vi "Taiko_LHDataToStrArray.vi"(11 "LHData":T2={"SerNo"=1034578, "Features"=16974033, "FreqMin"=1, "FreqMax"=100000000, "CwPowerMax"=77500000, "PulsePowerMax"=14500000, "WavelengthNominal"=6400, "CaseTempMax"=700, "Protection"=TRUE, "LHTypeCtrlVoltage"=4085, "LHMaxVoltage"=3590, "CurrentTEP12V"=100, "LaserType"=16, "LHVersion"={"Major"=0, "Minor"=0}, "CalWarrentHours"=1000} {"LaserType" items=["UNDEFINED"=0, "LDH"=16, "LDH_FSL"=24, "LED"=32, "TA_SHG"=48, "FIBER"=64, "FIBER_FSL"=72, "FA"=80, "FA_SHG"=96, "BRIDGE"=240]}) -> (3 "StrArray":string[](array[string]))   [LabVIEW 2019]
uses:
  <userlib>/TaikoLaser/PDLM_LHData.ctl
  <userlib>/TaikoLaser/PDLM_LHData_LaserType.ctl
  <userlib>/TaikoLaser/PDLM_LHVersion.ctl
panel:
  out "LaserType":T1 items=["UNDEFINED"=0, "LDH"=16, "LDH_FSL"=24, "LED"=32, "TA_SHG"=48, "FIBER"=64, "FIBER_FSL"=72, "FA"=80, "FA_SHG"=96, "BRIDGE"=240]
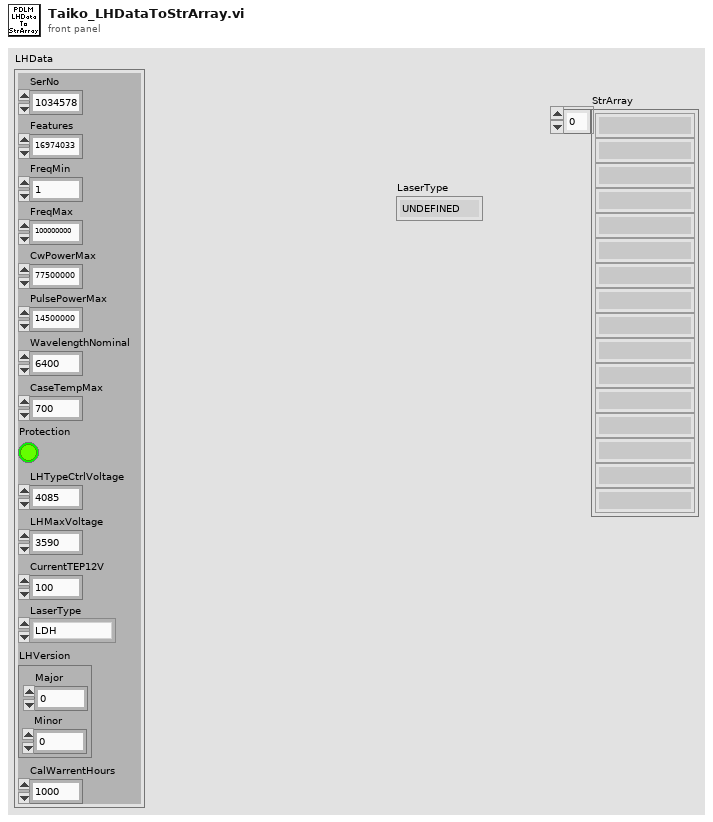
[diagram p1: front panel]
types:
  T1 = typedef "PDLM_LHData_LaserType.ctl" = u16
  T2 = typedef "PDLM_LHData.ctl" = cluster{"SerNo":u32, "Features":u32, "FreqMin":u32, "FreqMax":u32, "CwPowerMax":u32, "PulsePowerMax":u32, "WavelengthNominal":u16, "CaseTempMax":u16, "Protection":bool, "LHTypeCtrlVoltage":u16, "LHMaxVoltage":u16, "CurrentTEP12V":u16, "LaserType":T1, "LHVersion":T3, "CalWarrentHours":u16}
  T3 = typedef "PDLM_LHVersion.ctl" = cluster{"Major":u16, "Minor":u16}
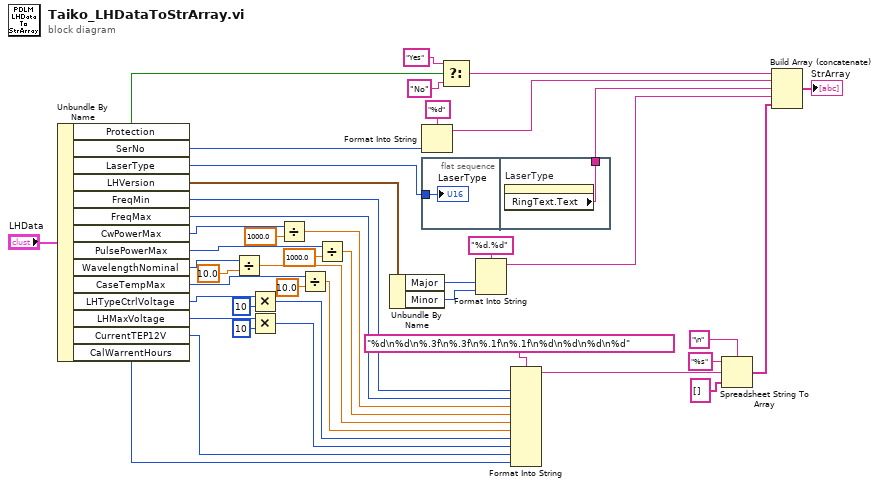
[diagram p0: block diagram]
diagram:
  n1 = Unbundle By Name("LHData") -> ("Protection"=w43:bool, "SerNo"=w40:u32, "LaserType"=w39:T1, "LHVersion"=w34:T3, "FreqMin"=w29:u32, "FreqMax"=w28:u32, "CwPowerMax"=w18:u32, "PulsePowerMax"=w14:u32, "WavelengthNominal"=w11:u16, "CaseTempMax"=w8:u16, "LHTypeCtrlVoltage"=w5:u16, "LHMaxVoltage"=w2:u16, "CurrentTEP12V"=w27:u16, "CalWarrentHours"=w26:u16)
  n2 = Divide(x=w11, y=10.0) -> (x/y=w10:dbl)
  n3 = Multiply(x=w5, y=u16 10) -> (x*y=w4:u16)
  n4 = Multiply(x=w2, y=u16 10) -> (x*y=w1:u16)
  n5 = Divide(x=w18, y=1000.0) -> (x/y=w16:dbl)
  n6 = Divide(x=w8, y=10.0) -> (x/y=w7:dbl)
  n7 = Divide(x=w14, y=1000.0) -> (x/y=w13:dbl)
  n8 = Unbundle By Name(w34) -> ("Major"=w33:u16, "Minor"=w32:u16)
  n9 = Format Into String(format string="%d", w40) -> (resulting string=w36:string)  [unwired: 2 in, 1 out]
  n10 = flat-sequence {
    tunnel: w39 -> [w45]
    tunnel: [w46] -> w35
    frame #0 {
      "LaserType" <- w45
    }
    frame #1 {
      n11 = property on="LaserType" class="MDér (strict)"() -> ("RingText.Text"=w46:string)  [unwired: 2 in, 2 out]
    }
  }
  n12 = Select(t="Yes", s=w43, f="No") -> (s? t:f=w37:string)
  n13 = Format Into String(format string="%d.%d", w33, w32) -> (resulting string=w30:string)  [unwired: 2 in, 1 out]
  n14 = Format Into String(format string="%d\n%d\n%.3f\n%.3f\n%.1f\n%.1f\n%d\n%d\n%d\n%d", w29, w28, w16, w13, w10, w7, w4, w1, w27, w26) -> (resulting string=w23:string)  [unwired: 2 in, 1 out]
  n15 = Spreadsheet String To Array(delimiter (Tab)="\n", format string="%s", spreadsheet string=w23, array type (2D Dbl)=string[] []) -> (array=w21:string[])
  n16 = Build Array (concatenate)(w37, w36, w35, w30, w21) -> (→"StrArray":string[])
